vi "Write ILC.vi"(10 "ILC":refnum<class "ILC.lvclass">, 11 "ILCDAC1 in":refnum<class "ILCDAC1.lvclass">) -> (3 "ILCDAC1 out":refnum<class "ILCDAC1.lvclass">)   [LabVIEW 2015, in "ILCDAC1.lvclass"]
uses:
  ILCDAC1.lvclass
  <userlib>/Common/ILC/ILC/ILC.lvclass
  ILCDAC1.lvclass/ILCDAC1.ctl
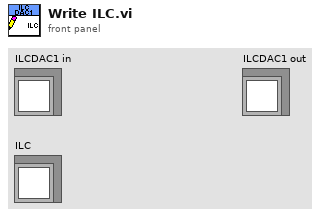
[diagram p1: front panel]
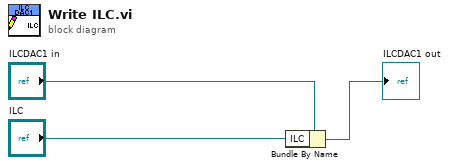
[diagram p0: block diagram]
diagram:
  n1 = Bundle By Name(cluster="ILCDAC1 in", "ILC"="ILC") -> (→"ILCDAC1 out":refnum<class "ILCDAC1.lvclass">)
